vi "Is Initialized.vi"(11 "Actor API in":refnum<class "Actor API.lvclass">) -> (2 "Initialized":bool)   [LabVIEW 2020, in "Artifex.lvlib" / "Actor API.lvclass"]
uses:
  Actor API.lvclass
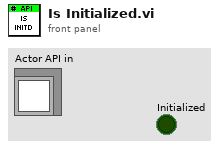
[diagram p1: front panel]
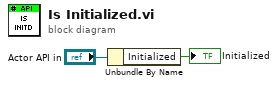
[diagram p0: block diagram]
diagram:
  n1 = Unbundle By Name("Actor API in") -> ("Initialized"=→"Initialized":bool)
